vi "ParseErrorCode.vi"(11 "String":string) -> (3 "number":i32[](array[numeric]))   [LabVIEW 2023]
uses:
  <vilib>/regexp/Match Regular Expression.xnode
panel:
  out "Array":string[](array[string])
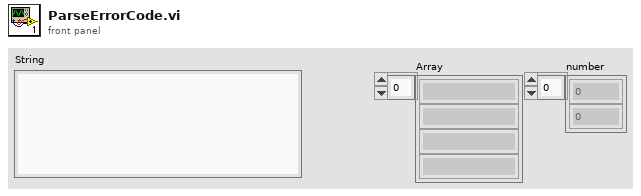
[diagram p1: front panel]
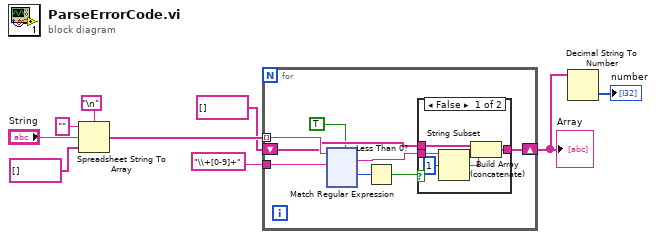
[diagram p0: block diagram]
diagram:
  n1 = Spreadsheet String To Array(delimiter (Tab)="\n", format string="", spreadsheet string="String", array type (2D Dbl)=string[] []) -> (array=w5:string[])
  n2 = for {
    tunnel: w5 -> [w17] mode=indexing
    tunnel: "\\+[0-9]+" ("regular expression") -> [w16]
    shift-right: [w14] -> w2
    shift-left: string[] [] ("Array") -> [w15]
    n3 = xnode "Match Regular Expression"("input string"=w17, "regular expression"=w16, "multiline? (F)"=TRUE) -> ("whole match"=w13:string, "offset past match"=w12:i32)  [unwired: 3 in, 3 out]
    n4 = Less Than 0?(x=w12) -> (x < 0?=w11:bool)
    n5 = case shown="False" w11 {
      tunnel: w15 -> [w22 w23]
      tunnel: w13 -> [w20 _]
      tunnel: [w21 w23] -> w14
      frame False {
        n6 = String Subset(string=w20, offset (0)=1) -> (substring=w19:string)  [unwired: 1 in]
        n7 = Build Array (concatenate)(w22, w19) -> (w21:string[])
      }
      frame True {
      }
    }
  }
  "Array" <- w2
  n8 = Decimal String To Number(string=w2) -> (number=→"number":i32[])  [unwired: 2 in, 1 out]
